vi "Aire5.vi"() -> ()   [LabVIEW 2023]
uses:
  <vilib>/MakerHub/LINX/LMH-LINX.lvlib
  <vilib>/MakerHub/LINX/Public/Peripherals/Analog/Analog Read 1 Chan.vi
  <vilib>/MakerHub/LINX/Public/Utilities/Open Serial.vi
  <vilib>/MakerHub/LINX/Public/Peripherals/Digital/Digital Write 1 Chan.vi
panel:
  out "Nivel Bajo":bool
  in  "stop":bool
  out "Nivel Alto":bool
  out "Smoke output":dbl(knob) scale=0.0..1025.0
  in  "Serial Port":refnum<visa-resource-name>="N/A"
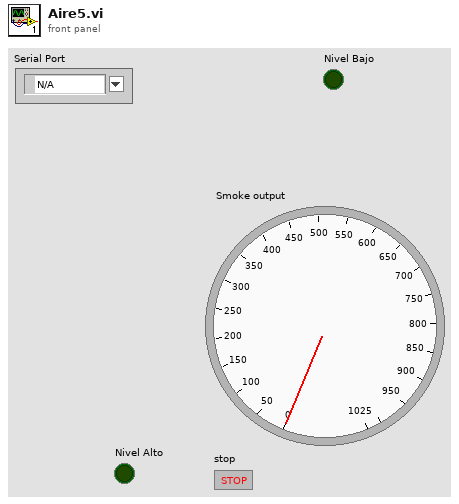
[diagram p1: front panel]
types:
  T1 = typedef "LMH-LINX.lvlib/LINX Ref.ctl" = cluster{"IO":T2, "Interface":T3, "LINX Device Config":T4}
  T2 = typedef "LMH-LINX.lvlib/Platform.ctl" = enum16{"Remote", "Local"}
  T3 = typedef "LMH-LINX.lvlib/Interface.ctl" = enum16{"Serial", "TCP"}
  T4 = typedef "LMH-LINX.lvlib/Device.lvlib/LINX Device Config.ctl" = cluster{"Interface":T3, "COM Port":refnum<visa-resource-name>, "TCP Configuration":T5, "Device Family":u8, "Device ID":u8, "Device Name":string, "TCP Ref":refnum<k5>, "Channels":T6}
  T5 = typedef "LMH-LINX.lvlib/Device.lvlib/TCP Config.ctl" = cluster{"IP Address":string, "Port":u16}
  T6 = typedef "LMH-LINX.lvlib/Channels.ctl" = cluster{"DI":u8[], "DO":u8[], "AI":u8[], "AO":u8[], "PWM":u8[], "QE":u8[], "UART":u8[], "I2C 2":u8[], "SPI":u8[], "CAN":u8[], "Servo":u8[], "AI Ref (V)":dbl, "AI Resolution (Bits)":u8, "AO Ref (V)":dbl, "AO Resolution (Bits)":u8}
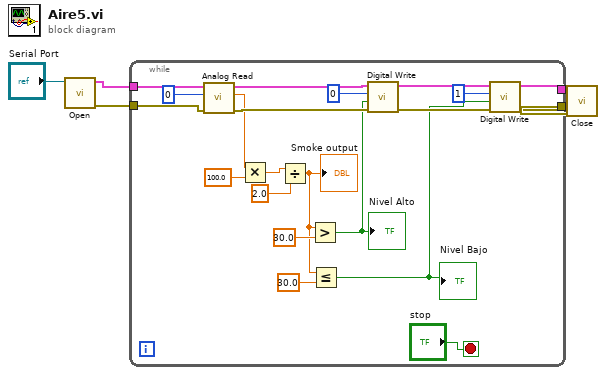
[diagram p0: block diagram]
diagram:
  n1 = call-poly <vilib>:"Open.vi"("Serial Port"="Serial Port") -> ("Error Out"=w3:errorcluster, "LINX Resource"=w2:T1)  [unwired: 8 in, 1 out]
  n2 = while {
    tunnel: [w9] -> w5
    tunnel: [w7] -> w4
    tunnel: w3 -> [w24]
    tunnel: w2 -> [w23]
    stop <- "stop" stop-if-true
    n3 = call-poly <vilib>:"Analog Read.vi"("Error In"=w24, "Analog Channel"=u8 0, "LINX Resource"=w23) -> ("Error Out"=w25:errorcluster, "Voltage"=w17:dbl, "LINX Resource"=w26:T1)  [unwired: 5 in, 1 out]
    n4 = Multiply(x=w17, y=100.0) -> (x*y=w16:dbl)
    n5 = Divide(x=w16, y=2.0) -> (x/y=w13:dbl)
    "Smoke output" <- w13
    n6 = Greater?(x=w13, y=30.0) -> (0:w20:bool)
    "Nivel Alto" <- w20
    n7 = Less Or Equal?(x=w13, y=30.0) -> (x <= y?=w6:bool)
    "Nivel Bajo" <- w6
    n8 = call-poly <vilib>:"Digital Write.vi"("Error In"=w25, "Output Value"=w20, "DO Channel"=u8 0, "LINX Resource"=w26) -> ("Error Out"=w8:errorcluster, "LINX Resource"=w10:T1)  [unwired: 6 in]
    n9 = call-poly <vilib>:"Digital Write.vi"("Error In"=w8, "Output Value"=w6, "DO Channel"=u8 1, "LINX Resource"=w10) -> ("Error Out"=w7:errorcluster, "LINX Resource"=w9:T1)  [unwired: 6 in]
  }
  n10 = call <vilib>:"Close.vi"("Error In"=w4, "LINX Resource"=w5) -> ()  [unwired: 9 in, 1 out]
